vi "Kddcup99.vi"(8 "error in (no error)":errorcluster caption="entrée d'erreur (pas d'erreur)", 11 "fetch_kddcup99":T2={"subset"="None", "shuffle"=TRUE, "random_state"=-1, "percent10"=TRUE, "download_if_missing"=TRUE, "Returns"="Data"} {"random_state" min=-1}) -> (0 "error out":errorcluster, 3 "Data":T1)   [LabVIEW 2020]
doc: "The KDD Cup ‘99 dataset was created by processing the tcpdump portions of the 1998 DARPA Intrusion Detection System (IDS) Evaluation dataset, created by MIT Lincoln Lab [1]. The artificial data (described on the dataset’s homepage) was generated using a closed network and hand-injected attacks to produce a large number of different types of attack with normal activity in the background. As the initial goal was to produce a large training set for supervised learning algorithms, there is a large proportion (80.1%) of abnormal data which is unrealistic in real world, and inappropriate for unsupervised anomaly detection which aims at detecting ‘abnormal’ data, ie\n 1 - qualitatively different from normal data\n 2 - in large minority among the observations.\nWe thus transform the KDD Data set into two different data sets: SA and SF.\n\n- SA is obtained by simply selecting all the normal data, and a small proportion of abnormal data to gives an anomaly proportion of 1%.\n\n- SF is obtained as in [2] by simply picking up the data whose attribute logged_in is positive, thus focusing on the intrusion attack, which gives a proportion of 0.3% of attack.\n\n- http and smtp are two subsets of SF corresponding with third feature equal to ‘http’ (resp. to ‘smtp’)\n\nGeneral KDD structure :\n\n - Samples total : 4898431\n - Dimensionality : 41\n - Features : discrete (int) or continuous (float)\n - Targets : str, ‘normal.’ or name of the anomaly type\nParameters :\n\n- subset : None, ‘SA’, ‘SF’, ‘http’, ‘smtp’\nTo return the corresponding classical subsets of kddcup 99. If None, return the entire kddcup 99 dataset.\n\n- shuffle : bool, default=False\nWhether to shuffle dataset.\n\n- random_state : int, RandomState instance, default=None=-1\nDetermines random number generation for dataset shuffling and for selection of abnormal samples if subset='SA'. Pass an int for reproducible output across multiple function calls. See Glossary.\n\n- percent10 : bool, default=True\nWhether to load only 10 percent of the data.\n\n- download_if_missing : bool, default=True\nIf False, raise a IOError if the data is not locally available instead of trying to download the data from the source site.\n\nReturns : \n\n- data : ndarray of shape (494021, 41)\nThe data matrix to learn.\n\n- target : ndarray of shape (494021,)\nThe regression target for each sample."
uses:
  Kddcup99.lvclass
panel:
  out "Kddcup99.lvclass":refnum<class "Kddcup99.lvclass">
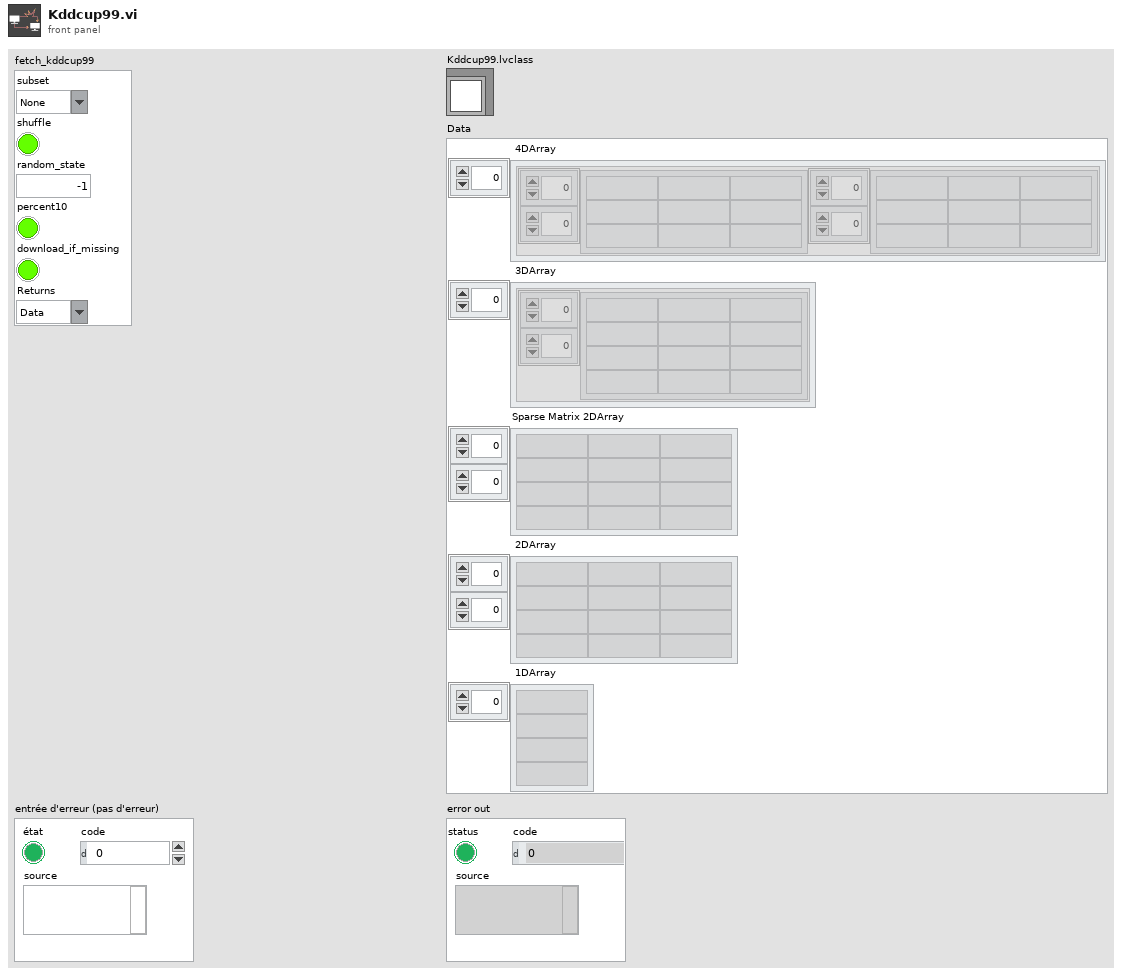
[diagram p1: front panel]
types:
  T1 = cluster{" 4DArray":cluster{"1":string[][], "2":string[][]}[], " 3DArray":cluster{"Tableau":string[][]}[], "Sparse Matrix 2DArray":string[][], " 2DArray":string[][], " 1DArray":string[]}
  T2 = cluster{"subset":string, "shuffle":bool, "random_state":i32, "percent10":bool, "download_if_missing":bool, "Returns":string}
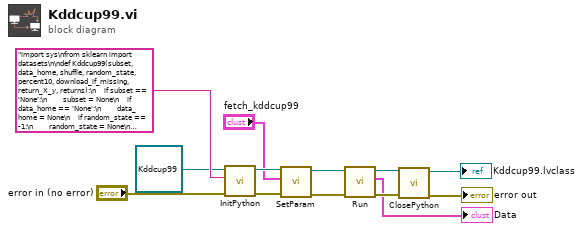
[diagram p0: block diagram]
diagram:
  n1 = call-dynamic "InitPython.vi"("error in (no error)"="error in (no error)", "Python Instruction"="import sys\nfrom sklearn import datasets\n\ndef Kddcup99(subset, data_home, shuffle, random_state, percent10, download_if_missing, return_X_y, returns):\n    if subset == 'None':\n        subset = None\n    if data_home == 'None':\n        data_home = None\n    if random_state == -1:\n        random_state = None\n    try:\n        Kddcup99 = datasets.fetch_kddcup99(subset, data_home, shuffle, random_state, percent10, download_if_missing, return_X_y)\n        if returns == 'Data': \n            data = Kddcup99['data'].tolist()\n            return str(data)\n        else :\n            data = Kddcup99['target'].tolist()\n            return str(data)\n    except:\n        erreur = sys.exc_info()\n        typerr = u\"%s\" % (erreur[0])\n        typerr = typerr[typerr.find(\"'\")+1:typerr.rfind(\"'\")]\n        msgerr = u\"%s\" % (erreur[1])\n        message = str('/!\\\\ {0} : {1}'. format(typerr,msgerr))\n        return message", "Scikit-learn en entrée"=refnum<class "Kddcup99.lvclass"> refnum ("Kddcup99.lvclass")) -> ("error out"=w9:errorcluster, "Scikit-learn en sortie"=w11:refnum<class "Kddcup99.lvclass">)  [unwired: 7 in]
  n2 = call-dynamic "SetParam.vi"("error in (no error)"=w9, "fetch_kddcup99"="fetch_kddcup99", "Kddcup99.lvclass"=w11) -> ("error out"=w6:errorcluster, "Kddcup99.lvclass"=w7:refnum<class "Kddcup99.lvclass">)  [unwired: 7 in]
  n3 = call-dynamic "Run.vi"("error in (no error)"=w6, "Kddcup99.lvclass"=w7) -> ("error in (no error)"=w4:errorcluster, "Data"=→"Data":T1, "Kddcup99.lvclass"=w5:refnum<class "Kddcup99.lvclass">)  [unwired: 7 in]
  n4 = call-dynamic "ClosePython.vi"("error in (no error)"=w4, "Scikit-learn en entrée"=w5) -> ("error out"=→"error out":errorcluster, "Scikit-learn en sortie"=→"Kddcup99.lvclass":refnum<class "Kddcup99.lvclass">)  [unwired: 8 in]
